vi "Charging_Gen Cals to Temp Set Points.vi"(8 "error in":errorcluster) -> (0 "error out":errorcluster, 1 "Abort Threshold (C)":dbl=nan format="%5.5f", 2 "Critical Threshold (C)":dbl=nan format="%5.5f", 3 "Warning Threshold (C)":dbl=nan format="%5.5f", 5 "Min Threshold (C)":dbl=nan format="%5.5f")   [LabVIEW 2010]
doc: "This function sends a Telemetry query to the IPG for General Calibration status including Temperature Thresholds (ohms). The Temperature Thresholds are converted from ohms to degrees Celsius.\n\nIf the status string format is incorrect, <not available> and NaN values will be returned."
uses:
  Telemetry/Typedef Command List.ctl
panel:
  out "Abort Threshold (ohms)":dbl=nan format="%.1f"
  out "Critical Threshold (ohms)":dbl=nan format="%.1f"
  out "Warning Threshold (ohms)":dbl=nan format="%.1f"
  out "Min Threshold (ohms)":dbl=nan format="%.1f"
  out "Gen Cals":string
  # "Get General Calibration\nfrom IPG"
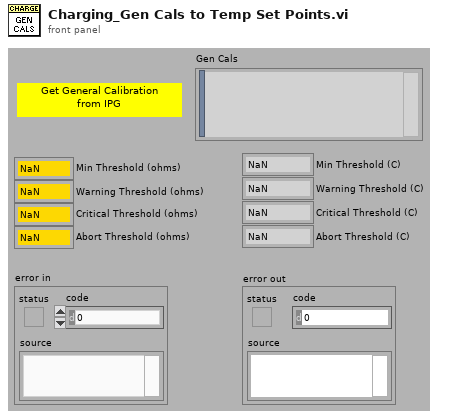
[diagram p1: front panel]
types:
  T1 = typedef "Typedef Command List.ctl" = enum16{"Get xPG Status", "xPG Stimulation", "Select Program", "Increment Program Amplitude", "Decrement Program Amplitude", "Get PoP Constants", "Get PPC Constants", "Get Program Names", "Set Pulse Amplitude", "Increment Pulse Amplitude", "Decrement Pulse Amplitude", "Get Pulse Widths", "Set Pulse Widths", "Increment Pulse Width", "Decrement Pulse Width", "Get Program Frequency", "Set Program Frequency", "Increment Program Frequency", "Decrement Program Frequency", "Inject Event", "Charging Control", "Get xPG Identity", "Set xPG Identity", "Restore Program Defaults", "Get Program Definition", "Set Program Definition", "Get Program Constants", "Set Program Constants", "Get Configurable Device Parameters", "Set Configurable Device Parameters", "Get Pulse Constants", "Set Pulse Constants", "Get Lead Limits", "Set Lead Limits", "Get Channel Calibrations", "Set Channel Calibrations", "<reserved 2>", "<reserved 3>", "<reserved 4>", "<reserved 5>", "<reserved 6>", "<reserved 7>", "Get Stim Asic HV Calibrations", "Set Stim Asic HV Calibrations", "<reserved 8>", "<reserved 9>", "Get CP Data", "Set CP Data", "Clear Log", "Read Log", "Append Log", "Get Patient Program Runtime", "Set Patient Program Runtime", "Impedance Measurement", "Enter Storage Mode", "Echo Short", "Echo Long", "Get General Calibration", "Set General Calibration", "Get Trim List", "Set Trim List", "Get Counter", "Set Counter", "Get Test Stimulation", "Set Test Stimulation", "Get Titration Stimulation", "Set Titration Stimulation", "Get Ramp Time", "Set Ramp Time", "Get VBAT", "Set Software Description Block", "Get Software Description Block", "Write Memory", "Read Memory", "Reset xPG", "Erase Flash Block", "Write Vectors", "Read Vectors", "Diagnostic Data", "Set Background Impedance", "Get Background Impedence ", "Set Test Waveform", "Calibrate Channel", "Get Log Range", "Reserved 0x55", "Reserved 0x56", "MICS Options", "Pair PPC", "Pair POP", "Stop Bootloader", "Tune MICS", "MICS Diagnostics", "Undefined"}
  T2 = cluster{"Command":T1, "Function":enum16{"Open Session", "Close Session", "Downlink Only", "Uplink Only", "Transceive (DN -> UP)"}, "MICS_ID":u32, "EXID":u32, "Use Local":bool, "Transceive Delay mS":dbl, "CP_DATA IN":u8[], "Parameters":string}
  T3 = enum16{"Open Session", "Close Session", "Downlink Only", "Uplink Only", "Transceive (DN -> UP)"}
  T4 = cluster{"Response Token":string, "Response Code":string, "bChecksum Valid":bool, "tChecksum Valid":bool, "CP_DATA OUT":u8[], "Data":string}
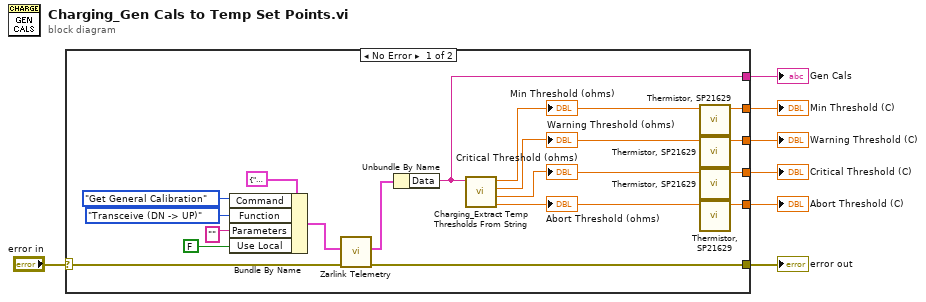
[diagram p0: block diagram]
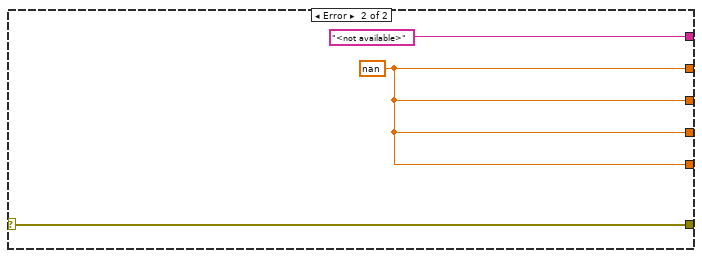
[diagram p2: hidden frame]
diagram:
  n1 = case shown="No Error" "error in" {
    selector: "error in" -> [w13 w26]
    tunnel: [w25 w26] -> w7
    tunnel: [w24 w27] -> w6
    tunnel: [w23 w27] -> w5
    tunnel: [w22 w27] -> w4
    tunnel: [w21 w27] -> w3
    tunnel: [w12 "<not available>" ("Data")] -> w1
    frame No Error {
      n2 = Bundle By Name(cluster=T2 {"Command"=enum."Get xPG Status", "Function"=enum."Close Session", "MICS_ID"=0, "EXID"=16773121, "Use Local"=FALSE, "Transceive Delay mS"=100.0, "CP_DATA IN"=[], "Parameters"=""} ("Input"), "Command"=Typedef_Command_List."Get General Calibration", "Function"=T3."Transceive (DN -> UP)", "Parameters"="", "Use Local"=FALSE) -> (w20:T2)
      n3 = call "Zarlink Telemetry.vi"("error in (no error)"=w13, "Input"=w20) -> ("error out"=w25:errorcluster, "Output"=w16:T4)  [unwired: 7 in, 1 out]
      n4 = Unbundle By Name(w16) -> ("Data"=w12:string)
      n5 = call "Charging_Extract Temp Thresholds From String.vi"("Gen Cals In"=w12) -> ("Abort Thresholdl (ohms)"=w8:dbl, "Critical Thresholdl (ohms)"=w9:dbl, "Warning Thresholdl (ohms)"=w10:dbl, "Min Threshold (ohms)"=w11:dbl)  [unwired: 7 in]
      "Min Threshold (ohms)" <- w11
      "Warning Threshold (ohms)" <- w10
      "Critical Threshold (ohms)" <- w9
      "Abort Threshold (ohms)" <- w8
      n6 = call "Thermistor, SP21629.vi"("resistance (ohms)"=w11) -> ("temperature (C)"=w24:dbl)  [unwired: 9 in, 1 out]
      n7 = call "Thermistor, SP21629.vi"("resistance (ohms)"=w10) -> ("temperature (C)"=w23:dbl)  [unwired: 9 in, 1 out]
      n8 = call "Thermistor, SP21629.vi"("resistance (ohms)"=w9) -> ("temperature (C)"=w22:dbl)  [unwired: 9 in, 1 out]
      n9 = call "Thermistor, SP21629.vi"("resistance (ohms)"=w8) -> ("temperature (C)"=w21:dbl)  [unwired: 9 in, 1 out]
    }
    frame Error {
      w27 = nan ("tempWarningThresholdl (ohms)")
    }
  }
  "error out" <- w7
  "Min Threshold (C)" <- w6
  "Warning Threshold (C)" <- w5
  "Critical Threshold (C)" <- w4
  "Abort Threshold (C)" <- w3
  "Gen Cals" <- w1
